vi "predict_extinction_angle.vi"() -> ()   [LabVIEW 2019]
panel:
  in  "m":dbl
  out "phi":dbl
  out "p hat parallel":dbl[](array[numeric])
  out "p hat perpendicular":dbl[](array[numeric])
  out "c hat":dbl[](array[numeric])
  out "Error Out":errorcluster
  in  "Error In":errorcluster
  in  "theta c":dbl
  in  "phi c":dbl
  out "phi_p_2":dbl
  out "phi_p_1":dbl
  in  "phi in":dbl
  in  "xi":dbl
  in  "gamma":dbl
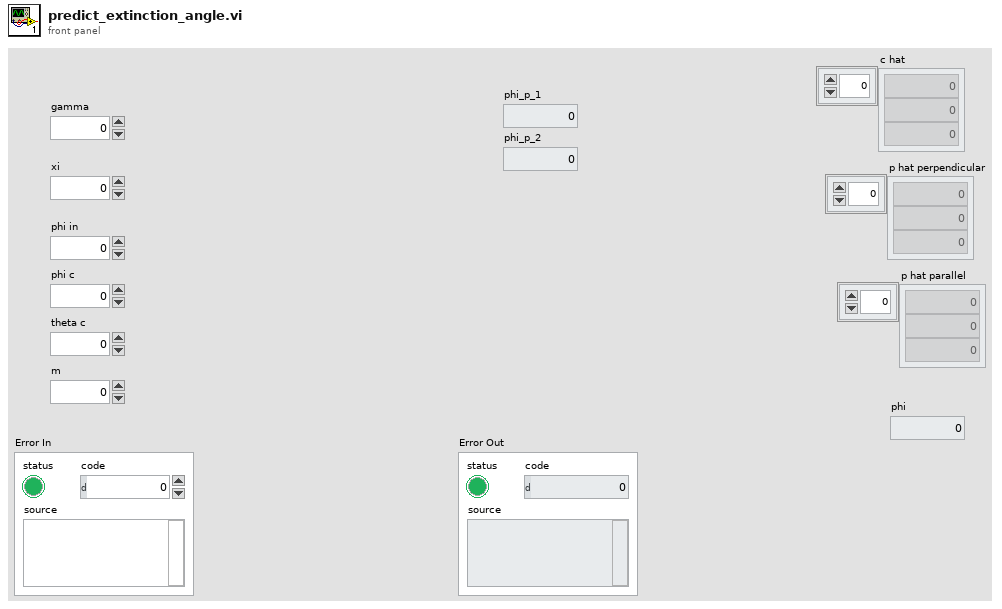
[diagram p1: front panel]
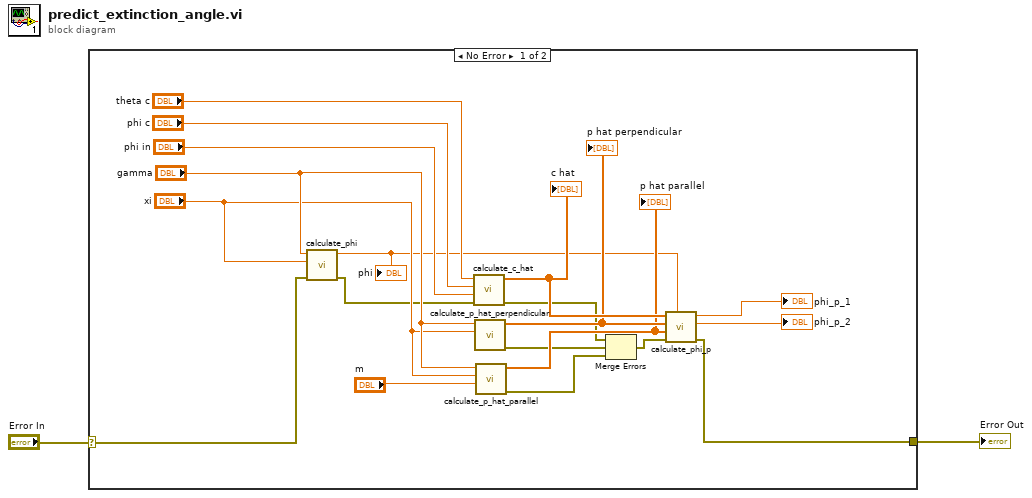
[diagram p0: block diagram]
diagram:
  n1 = case shown="No Error" "Error In" {
    selector: "Error In" -> [w6 w22]
    tunnel: [w5 w22] -> w1
    frame No Error {
      n2 = call "calculate_phi.vi"("Error In"=w6, "xi"="xi", "gamma"="gamma") -> ("Error Out"=w15:errorcluster, "phi"=w4:dbl)  [unwired: 7 in]
      "phi" <- w4
      n3 = call "calculate_c_hat.vi"("Error In"=w15, "phi_in"="phi in", "phi_c"="phi c", "theta_c"="theta c") -> ("Error Out"=w14:errorcluster, "c hat"=w21:dbl[])  [unwired: 6 in]
      "c hat" <- w21
      n4 = call "calculate_p_hat_perpendicular.vi"("xi"="xi", "gamma"="gamma") -> ("Error Out"=w13:errorcluster, "p hat perpendicular"=w20:dbl[])  [unwired: 8 in]
      "p hat perpendicular" <- w20
      n5 = call "calculate_p_hat_parallel.vi"("m"="m", "xi"="xi", "gamma"="gamma") -> ("Error Out"=w12:errorcluster, "p hat parallel"=w19:dbl[])  [unwired: 7 in]
      "p hat parallel" <- w19
      n6 = Merge Errors(w14, w13, w12) -> (w11:errorcluster)
      n7 = call "calculate_phi_p.vi"("phi"=w4, "Error In"=w11, "p_hat_parallel"=w19, "p_hat_perpendicular"=w20, "c_hat"=w21) -> ("Error Out"=w5:errorcluster, "phi_p_2"=→"phi_p_2":dbl, "phi_p_1"=→"phi_p_1":dbl)  [unwired: 4 in]
    }
    frame Error {
    }
  }
  "Error Out" <- w1
